vi "檢查落子.vi"(1 "Numeric 2":dbl, 2 "Numeric":dbl, 3 "フ":bool[][](array[boolean]), 4 "黑":bool[][](array[boolean])) -> (0 "黑 or 白？":bool)   [LabVIEW 2014]
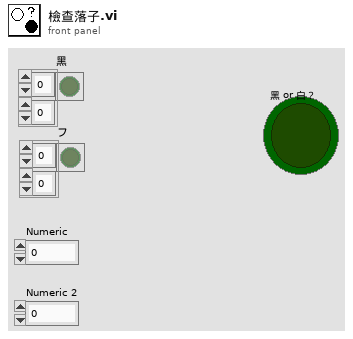
[diagram p1: front panel]
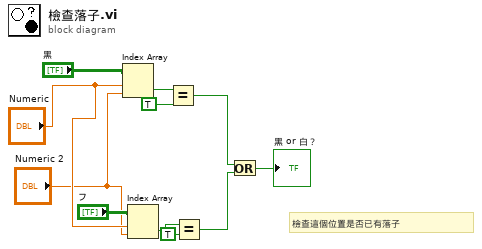
[diagram p0: block diagram]
diagram:
  # "檢查這個位置是否已有落子"
  n1 = Index Array(array="黑", index (row)="Numeric", index (col)="Numeric 2") -> (element=w7:bool)
  n2 = Index Array(array="フ", index (row)="Numeric", index (col)="Numeric 2") -> (element=w5:bool)
  n3 = Equal?(x=w7, y=TRUE) -> (x = y?=w3:bool)
  n4 = Equal?(x=w5, y=TRUE) -> (x = y?=w2:bool)
  n5 = Or(x=w3, y=w2) -> (x .or. y?=→"黑 or 白？":bool)
